vi "GetRAMValveState.vi"(7 "Timeout (ms)":u32=2000, 8 "Error In":errorcluster, 11 "Sierra M100 In":refnum<visa-resource-name>) -> (0 "Error Out":errorcluster, 2 "Valve State":T1, 3 "Sierra M100 Out":refnum<visa-resource-name>)   [LabVIEW 2012, in "Sierra-M100.lvlib"]
doc: "This VI gets the valve state from random access memory (RAM). RAM is volatile and the valve state is NOT retained during power cycling."
uses:
  Sierra-M100.lvlib
  Controls/ValveState.ctl
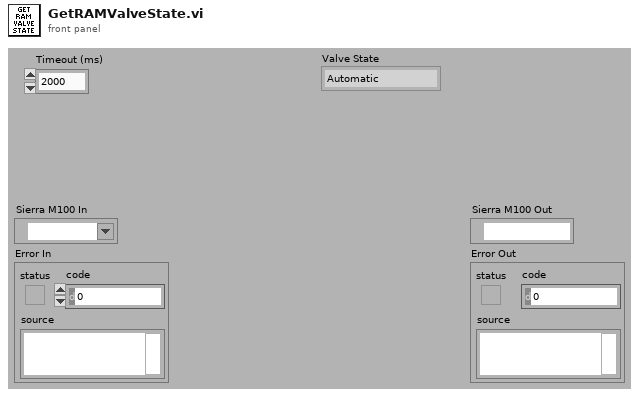
[diagram p1: front panel]
types:
  T1 = typedef "Sierra-M100.lvlib/ValveState.ctl" = enum16{"Automatic", "Closed", "Purge"}
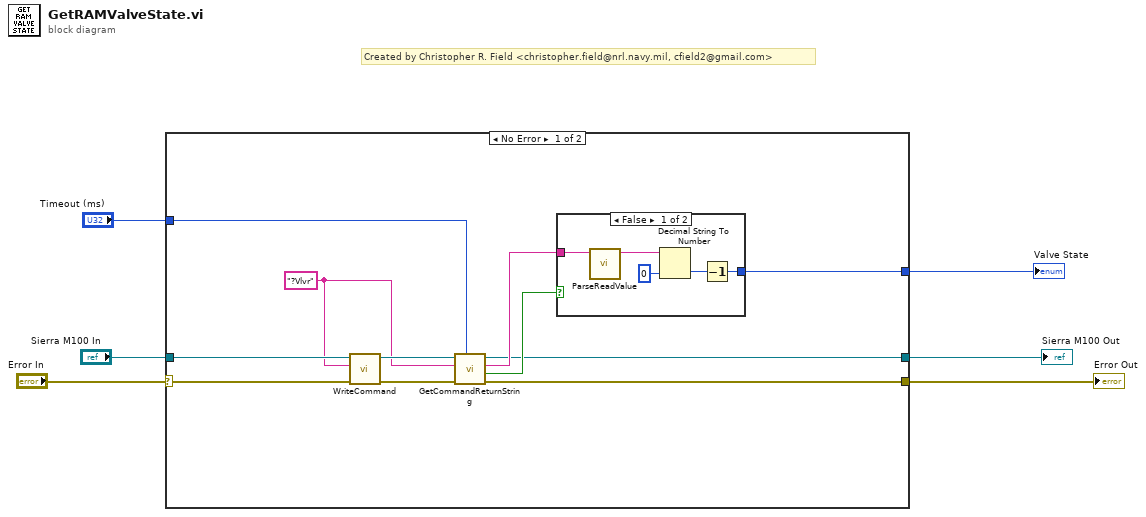
[diagram p0: block diagram]
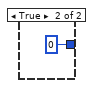
[diagram p2: hidden frame]
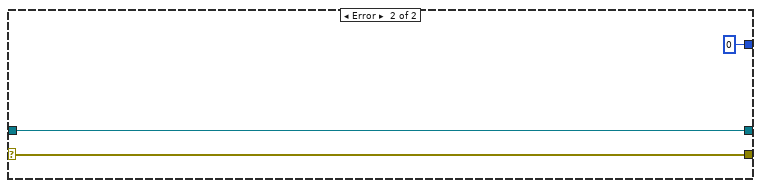
[diagram p3: hidden frame]
diagram:
  # "Created by Christopher R. Field <christopher.field@nrl.navy.mil, cfield2@gmail.com>"
  n1 = case shown="No Error" "Error In" {
    selector: "Error In" -> [w7 w25]
    tunnel: "Sierra M100 In" -> [w17 w26]
    tunnel: [w16 u16 0] -> w1
    tunnel: "Timeout (ms)" -> [w12 _]
    tunnel: [w9 w26] -> w4
    tunnel: [w8 w25] -> w3
    frame No Error {
      w13 = "?Vlvr"
      n2 = call "WriteCommand.vi"("Error In"=w7, "Command"=w13, "Sierra M100 In"=w17) -> ("Error Out"=w14:errorcluster, "Sierra M100 Out"=w15:refnum<visa-resource-name>)  [unwired: 5 in, 2 out]
      n3 = call "GetCommandReturnString.vi"("Timeout (ms)"=w12, "Error In"=w14, "Command"=w13, "Sierra M100 In"=w15) -> ("Error Out"=w8:errorcluster, "Timeout?"=w11:bool, "Return String"=w10:string, "Sierra M100 Out"=w9:refnum<visa-resource-name>)  [unwired: 4 in]
      n4 = case shown="False" w11 {
        tunnel: [w20 u16 0] -> w16
        tunnel: w10 -> [w18 _]
        frame False {
          n5 = call "ParseReadValue.vi"("Read Buffer"=w18) -> ("Value"=w19:string)  [unwired: 10 in]
          n6 = Decimal String To Number(string=w19, default (0L)=u16 0 ("default (0 I32)")) -> (number=w21:u16)  [unwired: 1 in, 1 out]
          n7 = Decrement(x=w21) -> (x-1=w20:u16)
        }
        frame True {
        }
      }
    }
    frame Error {
    }
  }
  "Sierra M100 Out" <- w4
  "Error Out" <- w3
  "Valve State" <- w1
